vi "Open.vi"() -> ()   [LabVIEW 2017]
uses:
  <vilib>/Instr/_visa.llb/VISA Configure Serial Port (Instr).vi
panel:
  in  "VISA resource name":refnum<visa-resource-name>="COM2"
  out "read buffer":string
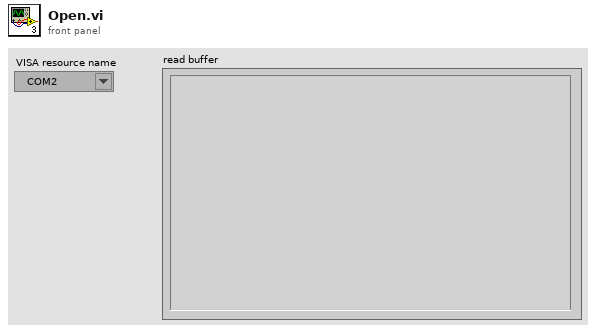
[diagram p1: front panel]
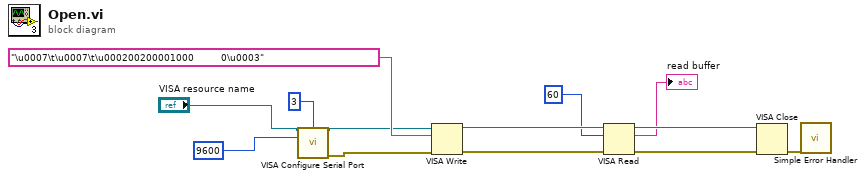
[diagram p0: block diagram]
diagram:
  n1 = call-poly "VISA Configure Serial Port"("VISA resource name"="VISA resource name", "termination char\n(0xA = '\\n' = LF)"=u8 3 ("termination char\n(0xA = '\\n' = LF)"), "baud rate (9600)"=u32 9600) -> ("VISA resource name out"=w4:refnum<visa-resource-name>, "error out"=w5:errorcluster)  [unwired: 11 in]
  n2 = VISA Write(VISA resource name=w4, write buffer="\u0007\t\u0007\t\u000200200001000         0\u0003", error in (no error)=w5) -> (VISA resource name out=w13:refnum<visa-resource-name>, error out=w12:errorcluster)  [unwired: 1 out]
  n3 = VISA Read(VISA resource name=w13, byte count=u32 60, error in (no error)=w12) -> (VISA resource name out=w10:refnum<visa-resource-name>, read buffer=→"read buffer":string, error out=w11:errorcluster)  [unwired: 1 out]
  n4 = VISA Close(VISA resource name=w10, error in (no error)=w11) -> (error out=w9:errorcluster)
  n5 = call <vilib>:"Simple Error Handler.vi"("error in (no error)"=w9) -> ()  [unwired: 4 in, 5 out]
